vi "Launch Nested Actors.vi"(8 "error in (no error)":errorcluster, 11 "Elevator Controller in":refnum<class "Elevator Controller.lvclass">) -> (0 "error out":errorcluster, 3 "Elevator Controller out":refnum<class "Elevator Controller.lvclass">)   [LabVIEW 2022 SP3, in "Elevator Controller.lvlib" / "Elevator Controller.lvclass"]
uses:
  Elevator Controller.lvclass
  Elevator Controller.lvclass/Elevator Controller.ctl
  <vilib>/ActorFramework/Actor/Actor.lvclass
  Sim User Console Actor/Abstract User Console Actor/Sim User Console Actor.lvclass
  Sim Display Console Actor/Sim Display Console Actor/Sim Display Console Actor.lvclass
  Sim Sensor Interface Actor/Sim Sensor Interface Actor/Sim Sensor Interface Actor.lvclass
  C:/Program Files/National Instruments/LabVIEW 2022/vi.lib/ActorFramework/Actor/Actor.lvclass
  C:/Workspace/CLA/Elevator AF_2022/Elevator Controller/Elevator Controller/Elevator Controller.lvclass
  Configuration Database Actor/Configuration Database Actor/Configuration Database Actor.lvclass
  C:/Workspace/CLA/Elevator AF_2022/Abstract User Console Actor/Abstract User Console Actor/Abstract User Console Actor.lvclass
  C:/Workspace/CLA/Elevator AF_2022/Sim User Console Actor/Abstract User Console Actor/Sim User Console Actor.lvclass
  C:/Workspace/CLA/Elevator AF_2022/Abstract Display Console/Abstract Display Console/Abstract Display Console.lvclass
  C:/Workspace/CLA/Elevator AF_2022/Sim Display Console Actor/Sim Display Console Actor/Sim Display Console Actor.lvclass
  C:/Workspace/CLA/Elevator AF_2022/Abstract Sensor Interface Actor/Abstract Sensor Interface Actor/Abstract Sensor Interface Actor.lvclass
  C:/Workspace/CLA/Elevator AF_2022/Sim Sensor Interface Actor/Sim Sensor Interface Actor/Sim Sensor Interface Actor.lvclass
  C:/Workspace/CLA/Elevator AF_2022/Configuration Database Actor/Configuration Database Actor/Configuration Database Actor.lvclass
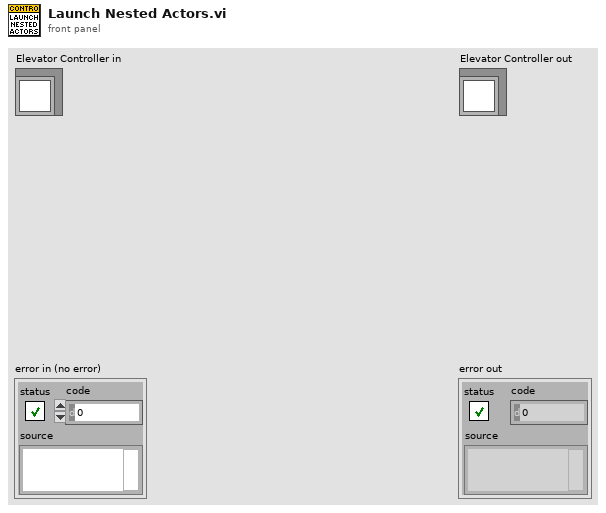
[diagram p1: front panel]
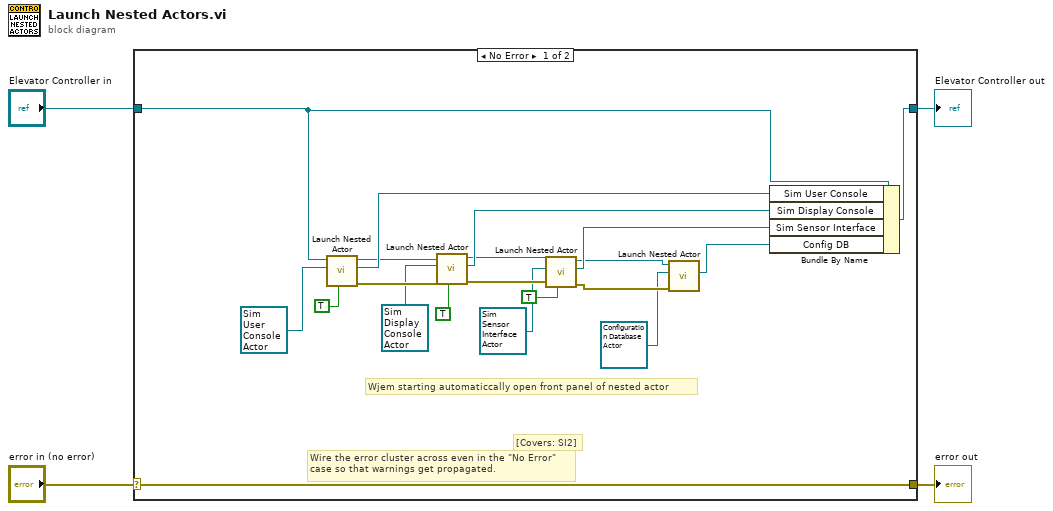
[diagram p0: block diagram]
diagram:
  n1 = case shown="No Error" "error in (no error)" {
    selector: "error in (no error)" -> [w24 w26]
    tunnel: [w24 w26] -> w3
    tunnel: [w20 w25] -> w1
    tunnel: "Elevator Controller in" -> [w22 w25]
    frame No Error {
      # "Wjem starting automaticcally open front panel of nested actor"
      # "[Covers: SI2]"
      # "Wire the error cluster across even in the \"No Error\"\ncase so that warnings get propagated."
      n2 = call <vilib>:"Launch Nested Actor.vi"("Open Actor Core front panel? (F)"=TRUE, "Nested Actor"=refnum<class "Sim User Console Actor.lvclass"> refnum ("Sim User Console Actor.lvlib:Sim User Console Actor.lvclass"), "Caller Actor in"=w22) -> ("error out"=w19:errorcluster, "Nested Actor's Enqueuer"=w21:refnum<class "Message Enqueuer.lvclass">, "Caller Actor out"=w18:refnum<class "Elevator Controller.lvclass">)  [unwired: 6 in]
      n3 = call <vilib>:"Launch Nested Actor.vi"("Open Actor Core front panel? (F)"=TRUE, "error in (no error)"=w19, "Nested Actor"=refnum<class "Sim Display Console Actor.lvclass"> refnum ("Sim Display Console Actor.lvlib:Sim Display Console Actor.lvclass"), "Caller Actor in"=w18) -> ("error out"=w12:errorcluster, "Nested Actor's Enqueuer"=w16:refnum<class "Message Enqueuer.lvclass">, "Caller Actor out"=w13:refnum<class "Elevator Controller.lvclass">)  [unwired: 5 in]
      n4 = call <vilib>:"Launch Nested Actor.vi"("Open Actor Core front panel? (F)"=TRUE, "error in (no error)"=w12, "Nested Actor"=refnum<class "Sim Sensor Interface Actor.lvclass"> refnum ("Sim Sensor Interface Actor.lvlib:Sim Sensor Interface Actor.lvclass"), "Caller Actor in"=w13) -> ("error out"=w7:errorcluster, "Nested Actor's Enqueuer"=w9:refnum<class "Message Enqueuer.lvclass">, "Caller Actor out"=w8:refnum<class "Elevator Controller.lvclass">)  [unwired: 5 in]
      n5 = call <vilib>:"Launch Nested Actor.vi"("error in (no error)"=w7, "Nested Actor"=refnum<class "Configuration Database Actor.lvclass"> refnum ("Configuration Database Actor.lvlib:Configuration Database Actor.lvclass"), "Caller Actor in"=w8) -> ("Nested Actor's Enqueuer"=w5:refnum<class "Message Enqueuer.lvclass">)  [unwired: 6 in, 2 out]
      n6 = Bundle By Name(cluster=w22, "Sim User Console"=w21, "Sim Display Console"=w16, "Sim Sensor Interface"=w9, "Config DB"=w5) -> (w20:refnum<class "Elevator Controller.lvclass">)
    }
    frame Error {
    }
  }
  "error out" <- w3
  "Elevator Controller out" <- w1
